vi "Random Square wave generator.vi"() -> ()   [LabVIEW 2023]
uses:
  <vilib>/measure/NI_MAPro.lvlib
  <vilib>/measure/mascope.llb/Transition Measurements 1 chan.vi
  <vilib>/measure/NI_MABase.lvlib
panel:
  out "Duration (low)":dbl
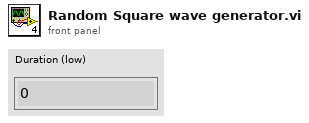
[diagram p1: front panel]
types:
  T1 = cluster{"start time":dbl, "end time":dbl, "ref levels":cluster{"high ref level":dbl, "mid ref level":dbl, "low ref level":dbl, "ref units":u16}}
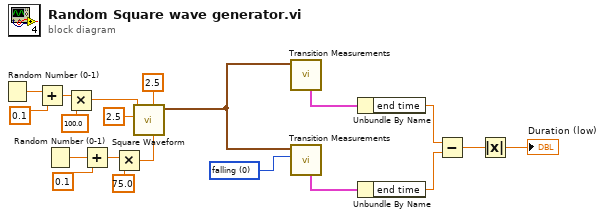
[diagram p0: block diagram]
diagram:
  w1 = u16 0 items=["falling", "rising"] ("polarity (rising)")
  n1 = Random Number (0-1)() -> (number: 0 to 1=w8:dbl)
  n2 = Add(x=w8, y=0.1) -> (x+y=w9:dbl)
  n3 = Random Number (0-1)() -> (number: 0 to 1=w6:dbl)
  n4 = Multiply(x=w9, y=100.0) -> (x*y=w12:dbl)
  n5 = Add(x=w6, y=0.1) -> (x+y=w5:dbl)
  n6 = Multiply(x=w5, y=75.0) -> (x*y=w3:dbl)
  n7 = call <vilib>:"Square Waveform.vi"("duty cycle (%)"=w3, "offset"=2.5, "amplitude"=2.5, "frequency"=w12) -> ("signal out"=w2:waveform(dbl))  [unwired: 6 in, 1 out]
  n8 = call-poly <vilib>:"Transition Measurements.vi"("signal in"=w2) -> ("measurement info"=w19:T1)  [unwired: 5 in, 5 out]
  n9 = call-poly <vilib>:"Transition Measurements.vi"("polarity (rising)"=w1, "signal in"=w2) -> ("measurement info"=w20:T1)  [unwired: 4 in, 5 out]
  n10 = Unbundle By Name(w19) -> ("end time"=w18:dbl)
  n11 = Unbundle By Name(w20) -> ("end time"=w17:dbl)
  n12 = Subtract(x=w18, y=w17) -> (x-y=w16:dbl)
  n13 = Absolute Value(x=w16) -> (abs(x)=→"Duration (low)":dbl)
